vi "Read Data.vi"(8 "Error In":errorcluster, 11 "Writer In":refnum<class "Writer.lvclass">) -> (0 "Error Out":errorcluster, 2 "Data":string, 3 "Writer Out":refnum<class "Writer.lvclass">)   [LabVIEW 2017, in "LabPack.lvlib" / "Writer.lvclass"]
uses:
  Writer.lvclass
  Writer.lvclass/Writer.ctl
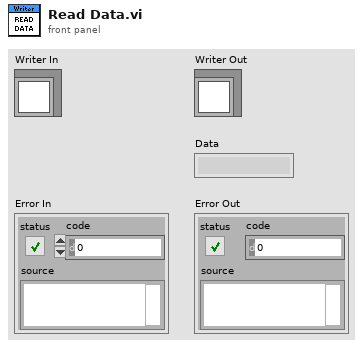
[diagram p1: front panel]
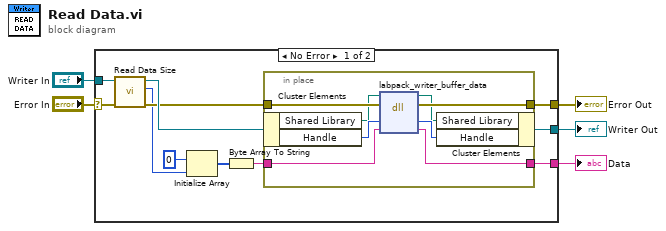
[diagram p0: block diagram]
diagram:
  n1 = case shown="No Error" "Error In" {
    selector: "Error In" -> [w13 w25]
    tunnel: "Writer In" -> [w14 w26]
    tunnel: [w15 w26] -> w3
    tunnel: [w16 w25] -> w2
    tunnel: [w6 _] -> w1
    frame No Error {
      n2 = call "Read Data Size.vi"("Error In"=w13, "Writer In"=w14) -> ("Error Out"=w11:errorcluster, "Data Size"=w9:u64, "Writer Out"=w12:refnum<class "Writer.lvclass">)  [unwired: 7 in]
      n3 = Initialize Array(u8 0, w9) -> (w8:u8[])
      n4 = Byte Array To String(unsigned byte array=w8) -> (string=w7:string)
      n5 = in-place {
        in-place-border: w11 -> [w24]
        in-place-border: [w23] -> w16
        in-place-border: w7 -> [w18]
        in-place-border: [w17] -> w6
        n6 = in-place-cluster #1(w12) -> ("Shared Library"=w20:path, "Handle"=w22:u64)
        n7 = dll-call lib="D:/Users/cfield/Code/MessagePack/LabPack/LabVIEW/trunk/src/LabPack/Private/labpack-x64.dll" fn="labpack_writer_buffer_data"(path in=w20, error in=w24, "writer"=w22, "buffer"=w18) -> (path out=w19:path, error out=w23:errorcluster, "writer"=w21:u64, "buffer"=w17:string)  [unwired: 2 in]
        n8 = in-place-cluster #1("Shared Library"=w19, "Handle"=w21) -> (w15:refnum<class "Writer.lvclass">)
      }
    }
    frame Error {
    }
  }
  "Writer Out" <- w3
  "Error Out" <- w2
  "Data" <- w1
